vi "2nd mom bg subtract.vi"(8 "error in (no error)":errorcluster, 9 "BG sub in":T1, 10 "2ndmom":T1, 11 "mask":T1) -> (0 "error out":errorcluster, 3 "thresh for 2nd mom out":T1)   [LabVIEW 2020, in "Point Grey Camera.lvclass"]
uses:
  Point Grey Camera.lvclass
  IMAQ Image.ctl
  NI_Vision_Development_Module.lvlib
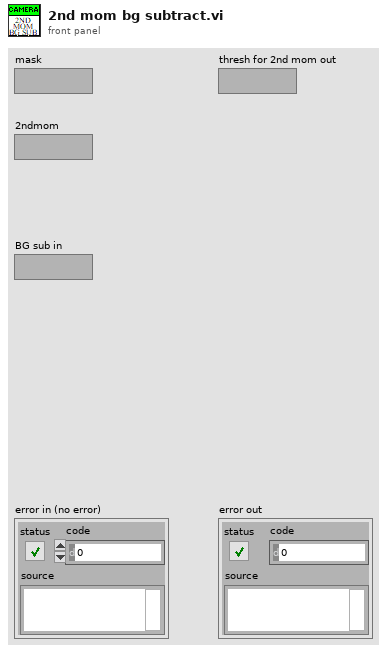
[diagram p1: front panel]
types:
  T1 = typedef "IMAQ Image.ctl" = refnum<image>
  T2 = typedef "ROI Descriptor" = cluster{"Global Rectangle":i32[], "Contours":cluster{"ID":enum32{"External", "Internal"}, "Type":u32, "Coordinates":i32[]}[]}
  T3 = cluster{"histogram":u32[], "Minimal Value":sgl, "Maximal Value":sgl, "Starting Value":sgl, "Interval Width":sgl, "Mean Value":sgl, "Standard  Variation":sgl, "Area (pixels)":i32}
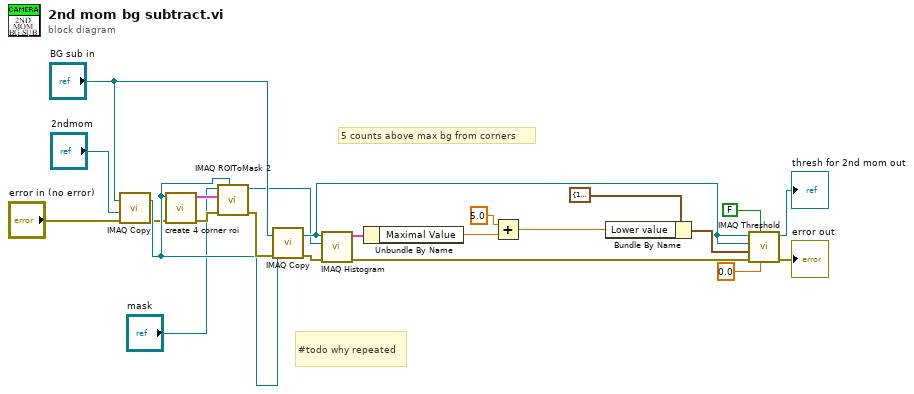
[diagram p0: block diagram]
diagram:
  # "#todo why repeated"
  # "5 counts above max bg from corners"
  n1 = call "IMAQ Copy"("error in (no error)"="error in (no error)", "Image Dst"="2ndmom", "Image Src"="BG sub in") -> ("error out"=w7:errorcluster, "Image Dst Out"=w8:T1)  [unwired: 3 in]
  n2 = call "create 4 corner roi.vi"("error in (no error)"=w7, "Refnum in"=w8) -> ("error out"=w3:errorcluster, "ROI Descriptor"=w4:T2)  [unwired: 8 in]
  n3 = call "IMAQ ROIToMask 2"("Image Model"=w8, "error in (no error)"=w3, "ROI Descriptor"=w4, "Image"="mask") -> ("error out"=w10:errorcluster, "Image Out"=w11:T1)  [unwired: 5 in, 1 out]
  n4 = call "IMAQ Copy"("error in (no error)"=w10, "Image Dst"=w8, "Image Src"="BG sub in") -> ("error out"=w22:errorcluster, "Image Dst Out"=w21:T1)  [unwired: 3 in]
  n5 = call "IMAQ Histogram"("error in (no error)"=w22, "Image Mask"=w11, "Image"=w21) -> ("error out"=w20:errorcluster, "Histogram Report"=w15:T3)  [unwired: 7 in]
  n6 = Unbundle By Name(w15) -> ("Maximal Value"=w14:sgl)
  n7 = Add(x=sgl 5.0, y=w14) -> (x+y=w13:sgl)
  n8 = Bundle By Name(cluster=cluster{"Lower value":sgl, "Upper value":sgl} {"Lower value"=100.0, "Upper value"=9999999.0} ("Range"), "Lower value"=w13) -> (w16:cluster{"Lower value":sgl, "Upper value":sgl})
  n9 = call "IMAQ Threshold"("Replace Value"=sgl 0.0, "Keep/Replace Value (Replace)"=FALSE, "error in (no error)"=w20, "Range"=w16, "Image Dst"=w21, "Image Src"=w21) -> ("error out"=→"error out":errorcluster, "Image Dst Out"=→"thresh for 2nd mom out":T1)  [unwired: 4 in]
